vi "Self Event Alias.vi"(11 "Template Event in":refnum<class "Template Event.lvclass">) -> (2 "Self Event Alias":string)   [LabVIEW 2021, in "_Template.lvlib" / "Templates.lvlib" / "Template Event.lvlib" / "Template Event.lvclass"]
uses:
  Template Event.lvclass
  Template Event.lvclass/Template Event.ctl
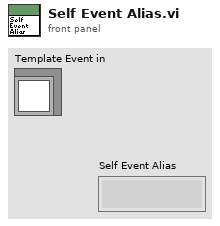
[diagram p1: front panel]
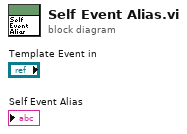
[diagram p0: block diagram]
diagram:
